vi "Initialize Array Activity.vi"() -> ()   [LabVIEW 2012]
panel:
  out "?":dbl[][](array[numeric])
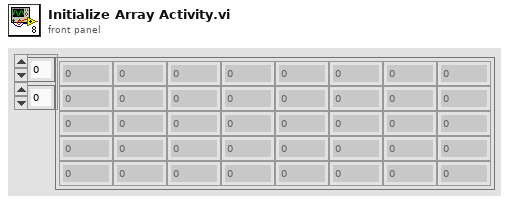
[diagram p1: front panel]
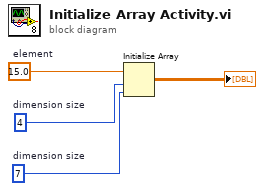
[diagram p0: block diagram]
diagram:
  w2 = 7  # dimension size
  w3 = 4  # dimension size
  w4 = 15.0  # element
  n1 = Initialize Array(w4, w3, w2) -> (→"?":dbl[][])
